vi "Value Has Changed String PtByPt.vi"(0 "input data point":string, 1 "initialize":bool) -> (2 "has changed":bool, 3 "output data point":string)   [LabVIEW 2015]
doc: "Detects changes of <B>input data point</B> between the current call and the previous call to the Value Has Changed PtByPt VI."
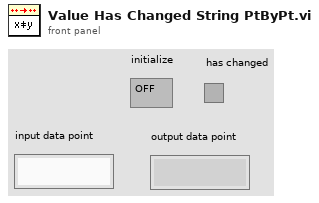
[diagram p1: front panel]
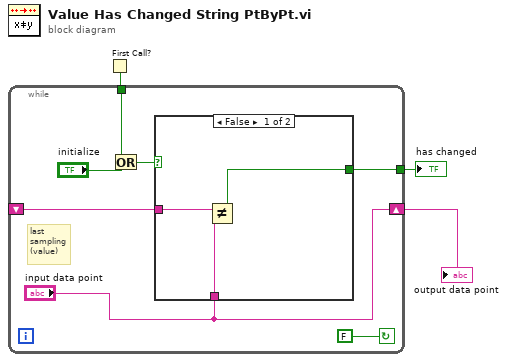
[diagram p0: block diagram]
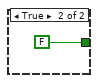
[diagram p2: hidden frame]
diagram:
  n1 = First Call?() -> (First Call?: T/F=w2:bool)
  n2 = while {
    tunnel: w2 -> [w5]
    tunnel: [w10] -> w3
    shift-left: _ -> [w9]
    shift-right: ["input data point"] -> w1
    stop <- FALSE continue-if-true
    # "last\nsampling\n(value)"
    n3 = Or(x=w5, y="initialize") -> (x .or. y?=w7:bool)
    n4 = case shown="False" w7 {
      tunnel: [w11 FALSE] -> w10
      tunnel: w9 -> [w13 _]
      tunnel: "input data point" -> [w12 _]
      frame False {
        n5 = Not Equal?(x=w13, y=w12) -> (x != y?=w11:bool)
      }
      frame True {
      }
    }
  }
  "has changed" <- w3
  "output data point" <- w1
